vi "Enqueue Message (Single).vi"(6 "Priority Message? (F)":bool, 8 "error in (no error)":errorcluster, 9 "Message Data":variant, 10 "Message":string, 11 "Message Queue":refnum<queue>) -> (0 "error out":errorcluster, 3 "dup Message Queue":refnum<queue>)   [LabVIEW 2017, in "Message Queue.lvlib"]
doc: "For a regular message, enqueue the message. For a priority message, enqueue it at the front of the queue."
uses:
  Message Queue.lvlib
  Message Cluster.ctl
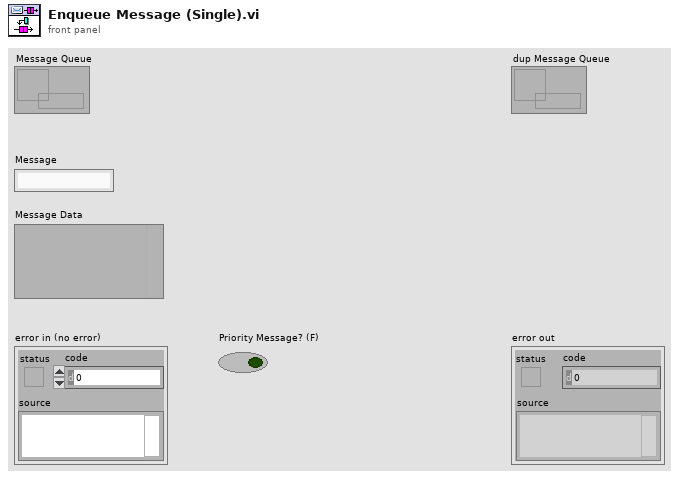
[diagram p1: front panel]
types:
  T1 = typedef "Message Queue.lvlib/Message Cluster.ctl" = cluster{"Message":string, "Message Data":variant}
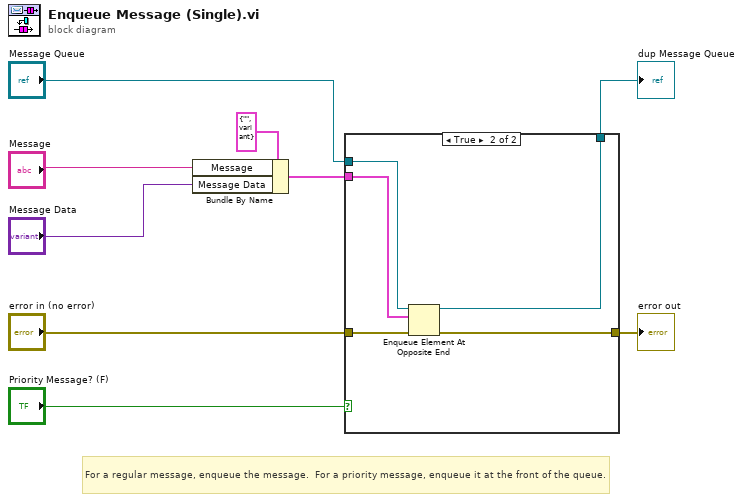
[diagram p0: block diagram]
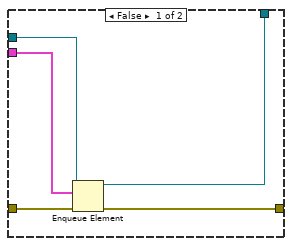
[diagram p2: hidden frame]
diagram:
  # "For a regular message, enqueue the message.  For a priority message, enqueue it at the front of the queue."
  n1 = Bundle By Name(cluster=T1 {"Message"="", "Message Data"=variant} ("Message Cluster"), "Message"="Message", "Message Data"="Message Data") -> (w3:T1)
  n2 = case shown="True" "Priority Message? (F)" {
    tunnel: "error in (no error)" -> [w14 w19]
    tunnel: [w13 w18] -> w4
    tunnel: "Message Queue" -> [w10 w17]
    tunnel: w3 -> [w12 w16]
    tunnel: [w11 w15] -> w1
    frame False {
      n3 = Enqueue Element(queue=w10, element=w12, error in (no error)=w14) -> (queue out=w11:refnum<queue>, error out=w13:errorcluster)  [unwired: 1 in, 1 out]
    }
    frame True {
      n4 = Enqueue Element At Opposite End(queue=w17, element=w16, error in (no error)=w19) -> (queue out=w15:refnum<queue>, error out=w18:errorcluster)  [unwired: 1 in, 1 out]
    }
  }
  "error out" <- w4
  "dup Message Queue" <- w1
